vi "ScoreEntry.vi"(7 "LabVIEW Web Service Request":refnum<class "Web Request.lvclass">) -> ()   [LabVIEW 2013]
uses:
  <vilib>/wsapi/Web Request.lvclass
  <vilib>/Utility/sysdir.llb/System Directory Type.ctl
panel:
  # "Use the Web Service Request input terminal to call the VIs on the Web Services palette. Do not remove it from the connector pane unless you don't need access to the palette."
  # "Each additional control wired to the connector pane will be available as an input in the URL. To include an indicator in terminal-mode output (the default setting), it must also be wired to the connector pane."
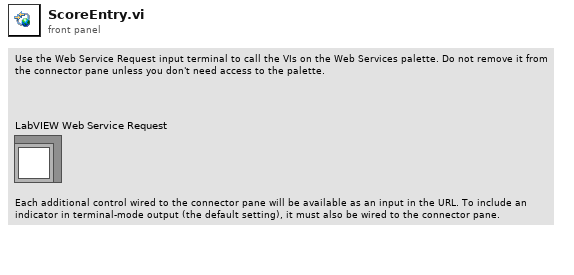
[diagram p1: front panel]
types:
  T1 = typedef "System Directory Type.ctl" = i32
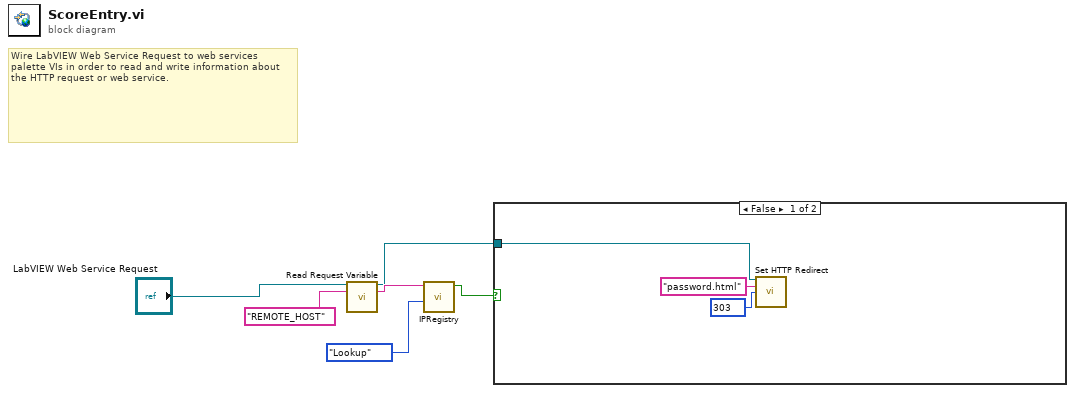
[diagram p0: block diagram]
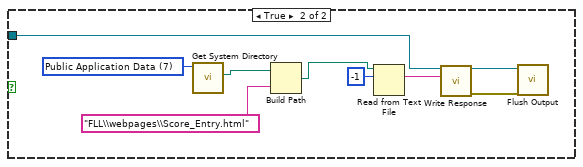
[diagram p2: hidden frame]
diagram:
  # "Wire LabVIEW Web Service Request to web services palette VIs in order to read and write information about the HTTP request or web service."
  n1 = call <vilib>:"Read Request Variable.vi"("LabVIEW Web Service Request"="LabVIEW Web Service Request", "variable name"="REMOTE_HOST") -> ("LabVIEW Web Service Request out"=w1:refnum<class "Web Request.lvclass">, "value"=w4:string)  [unwired: 11 in, 1 out]
  n2 = call "IPRegistry.vi"("Action"=enum16{"Flush All", "Lookup", "Add"}."Lookup", "IP Address"=w4) -> ("Success"=w2:bool)  [unwired: 8 in, 1 out]
  n3 = case shown="False" w2 {
    tunnel: w1 -> [w9 w10]
    frame False {
      w7 = 303 items=["100"=100, "101"=101, "200"=200, "201"=201, "202"=202, "203"=203, "204"=204, "205"=205, "206"=206, "300"=300, "301"=301, "302"=302, "303"=303, "304"=304, "305"=305, "306"=306, "307"=307, "400"=400, "401"=401, "402"=402, "403"=403, "404"=404, "405"=405, "406"=406, "407"=407, "408"=408, "409"=409, "410"=410, "411"=411, "412"=412, "413"=413, "414"=414, "415"=415, "416"=416, "417"=417, "500"=500, "501"=501, "502"=502, "503"=503, "504"=504, "505"=505] ("response code (307)")
      n4 = call <vilib>:"Set HTTP Redirect.vi"("LabVIEW Web Service Request"=w9, "redirect URL"="password.html", "response code (307)"=w7) -> ()  [unwired: 11 in, 2 out]
    }
    frame True {
      w11 = T1 7 items=["User Home"=0, "User Desktop"=1, "User Documents"=2, "User Application Data"=3, "User Preferences"=4, "User Temporary"=5, "Public Documents"=6, "Public Application Data"=7, "Public Preferences"=8, "Public Cache"=13, "System Core Libraries"=9, "System Installed Libraries"=10, "Application Files"=11, "Boot Volume Root"=12] ("system directory type")
      n5 = call <vilib>:"Get System Directory.vi"("system directory type"=w11) -> ("system directory"=w13:path)  [unwired: 10 in]
      n6 = Build Path(base path=w13, name or relative path="FLL\\webpages\\Score_Entry.html") -> (appended path=w15:path)
      n7 = Read from Text File(file (use dialog)=w15, count=-1) -> (text=w18:string)  [unwired: 2 in, 3 out]
      n8 = call <vilib>:"Write Response.vi"("LabVIEW Web Service Request"=w10, "response string"=w18) -> ("LabVIEW Web Service Request out"=w16:refnum<class "Web Request.lvclass">, "error out"=w17:errorcluster)  [unwired: 12 in]
      n9 = call <vilib>:"Flush Output.vi"("LabVIEW Web Service Request"=w16, "error in (no error)"=w17) -> ()  [unwired: 12 in, 2 out]
    }
  }
